vi "Waveform Chart.vi"() -> ()   [LabVIEW 2019]
panel:
  out "Waveform Chart":cluster{i32, i32, i32, i32}[](graph)
  out "Waveform Chart 2":i32[][](graph)
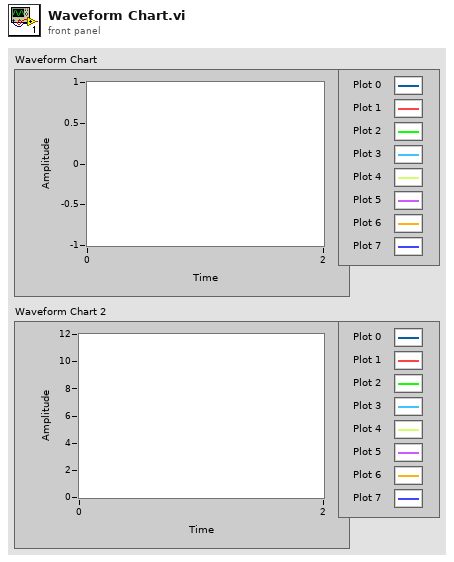
[diagram p1: front panel]
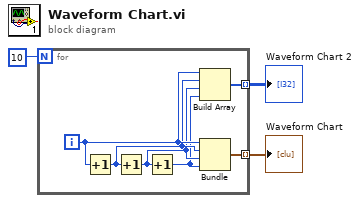
[diagram p0: block diagram]
diagram:
  n1 = for {
    N: 10 -> [_]
    tunnel: [w5] -> w2 mode=indexing
    tunnel: [w4] -> w1 mode=indexing
    i -> [w9]
    n2 = Increment(x=w9) -> (x+1=w8:i32)
    n3 = Increment(x=w8) -> (x+1=w7:i32)
    n4 = Increment(x=w7) -> (x+1=w6:i32)
    n5 = Build Array(w9, w8, w7, w6) -> (w5:i32[])
    n6 = Bundle(w9, w8, w7, w6) -> (w4:cluster{i32, i32, i32, i32})  [unwired: 1 in]
  }
  "Waveform Chart" <- w1
  "Waveform Chart 2" <- w2
